vi "BoundAngle.vi"(1 "Type":T1(ring), 2 "Angle":dbl) -> (0 "Bound Angle":dbl)   [LabVIEW 2016]
doc: "Help by FRC Team 836 - The RoboBees\nVI takes an angle input and depending on selected funtion either:\n1. The portion of the input between 0 and 360 degrees\n2. The angle between either -180 or 180 degrees\n3. The portion of the angle between 0 and 2Pi radians\n4. The angle between -Pi and Pi radians"
panel:
  # "Help by FRC Team 836 - The RoboBees\nVI takes an angle input and depending on selected funtion either:\n1.  The portion of the input between 0 and 360 degrees\n2.  The angle between either -180 or 180 degrees\n3.  The portion of the angle between 0 and 2Pi radians\n4.  The angle between -Pi and Pi radians"
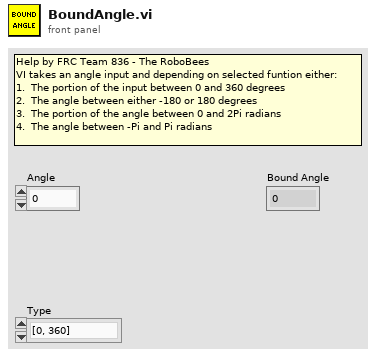
[diagram p1: front panel]
types:
  T1 = enum16{"[0, 360]", "[-180, 180]", "[0, 2PI]", "[-PI, PI]"}
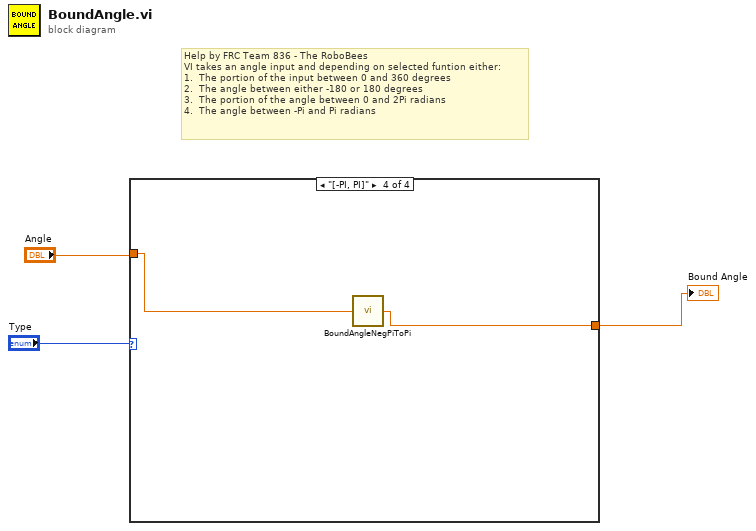
[diagram p0: block diagram]
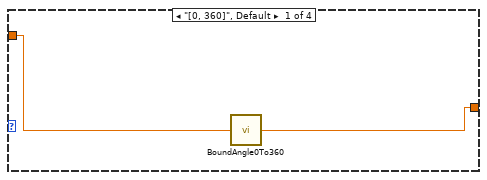
[diagram p2: hidden frame]
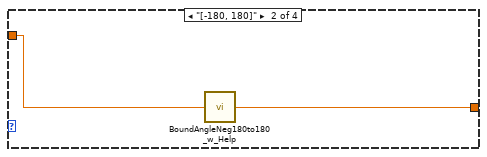
[diagram p3: hidden frame]
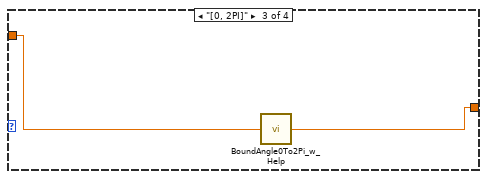
[diagram p4: hidden frame]
diagram:
  # "Help by FRC Team 836 - The RoboBees\nVI takes an angle input and depending on selected funtion either:\n1.  The portion of the input between 0 and 360 degrees\n2.  The angle between either -180 or 180 degrees\n3.  The portion of the angle between 0 and 2Pi radians\n4.  The angle between -Pi and Pi radians"
  n1 = case shown="\"[-PI, PI]\"" "Type" {
    tunnel: "Angle" -> [w5 w7 w9 w11]
    tunnel: [w4 w6 w8 w10] -> w1
    frame "[0, 360]", Default {
      n2 = call <userlib>:"BoundAngle0To360.vi"("angle"=w5) -> ("bound angle"=w4:dbl)
    }
    frame "[-180, 180]" {
      n3 = call <userlib>:"BoundAngleNeg180to180_w_Help.vi"("angle"=w7) -> ("bound angle"=w6:dbl)
    }
    frame "[0, 2PI]" {
      n4 = call <userlib>:"BoundAngle0To2Pi_w_Help.vi"("angle"=w9) -> ("bound angle"=w8:dbl)
    }
    frame "[-PI, PI]" {
      n5 = call <userlib>:"BoundAngleNegPiToPi.vi"("angle"=w11) -> ("bound angle"=w10:dbl)
    }
  }
  "Bound Angle" <- w1
